vi "readFromFile.vi"(11 "file path (dialog if empty)":path) -> (3 "data":dbl[](array[numeric]))   [LabVIEW 2016]
uses:
  <vilib>/Utility/file.llb/Read Delimited Spreadsheet (DBL).vi
panel:
  out "all rows":dbl[][](array[numeric])
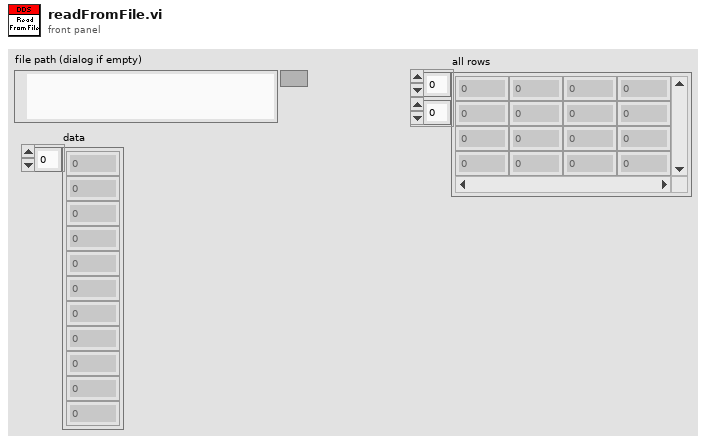
[diagram p1: front panel]
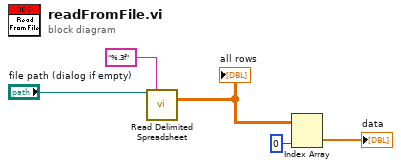
[diagram p0: block diagram]
diagram:
  n1 = call-poly <vilib>:"Read Delimited Spreadsheet.vi"("file path (dialog if empty)"="file path (dialog if empty)", "format (%.3f)"="%.3f") -> ("all rows"=w1:dbl[][])  [unwired: 8 in, 5 out]
  "all rows" <- w1
  n2 = Index Array(array=w1, index (col)=0 ("disabled index (col)")) -> (element=→"data":dbl[])  [unwired: 1 in]
